vi "proceso1.vi"() -> ()   [LabVIEW 2020]
panel:
  out "proceso1":T1
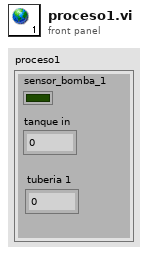
[diagram p1: front panel]
types:
  T1 = cluster{"sensor_bomba_1":bool, "tanque in":u8, " tuberia 1":u8}
diagram:
